vi "mqtt client server.vi"(6 "keep connected":refnum<vi>, 8 "connect success reference":refnum<vi>, 9 "mqtt prefix":string, 10 "client or server":enum16{"client", "server"}(ring), 11 "subsystem":string) -> (0 "error out":errorcluster)   [LabVIEW 2017]
uses:
  mqtt-LabVIEW/src/class/mqtt/mqttTypedef/mqttBroker.ctl
  mqtt-LabVIEW/src/class/mqtt/mqttTypedef/mqttConnectionFlags.ctl
  mqtt-LabVIEW/src/class/mqtt/mqttTypedef/mqttUserInformation.ctl
  mqtt-LabVIEW/src/class/mqtt/mqttTypedef/mqttWillInformation.ctl
  mqtt-LabVIEW/src/class/mqtt/mqttConfigFunction.ctl
  mqtt-LabVIEW/src/class/mqtt/mqttTXqueue/mqttTXdataQueueFunction.ctl
  mqtt-LabVIEW/src/class/mqtt/mqtt.lvclass
panel:
  out "connect success":bool
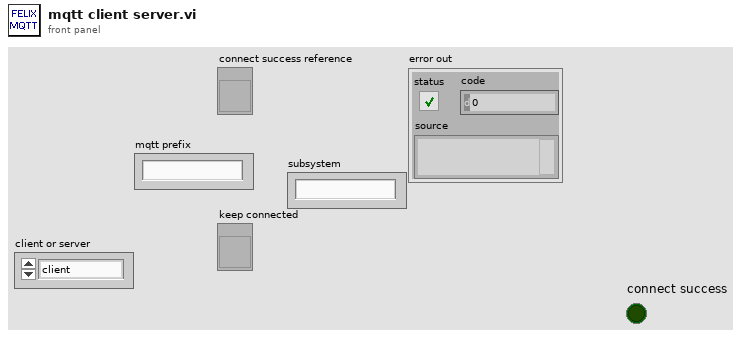
[diagram p1: front panel]
types:
  T1 = typedef "mqttWillInformation.ctl" = cluster{"User Name":string, "Password":string}
  T2 = typedef "mqttUserInformation.ctl" = cluster{"Will message":string, "Will Topic":string}
  T3 = typedef "mqttConnectionFlags.ctl" = cluster{"reserved":bool, "clean session":bool, "will flag":bool, "willQOS":enum8{"At most once", "At least once", "Exactly once", "Reserved"}, "will retain":bool, "password":bool, "user name":bool}
  T4 = typedef "mqttBroker.ctl" = cluster{"address":string, "port":u16, "connTimeout":i32, "writeTimeout":i32, "readTimeout":i32, "subTimeout":i32}
  T5 = typedef "mqttTXdataQueueFunction.ctl" = enum16{"init", "deinit", "getQueue", "enqueue"}
  T6 = typedef "mqtt.lvclass/mqttConfigFunction.ctl" = enum16{"init", "deinit", "set", "get"}
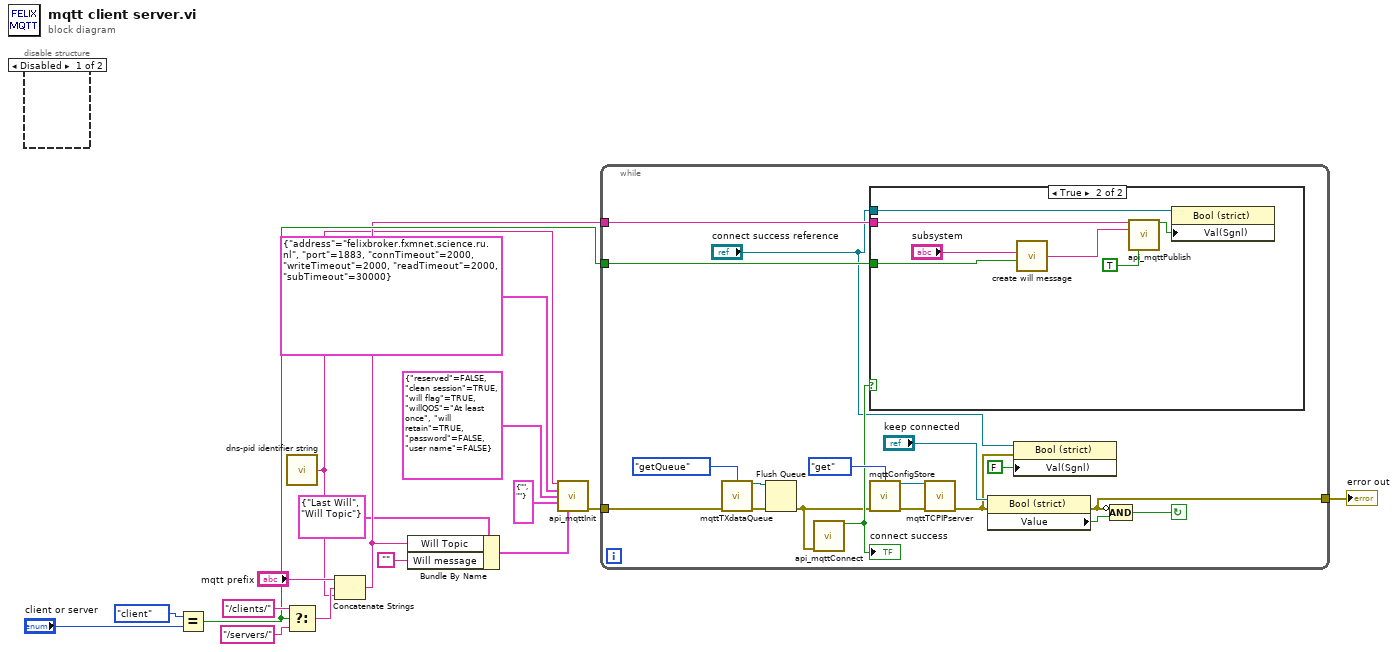
[diagram p0: block diagram]
diagram:
  n1 = disable-structure shown="Disabled" {
    frame Disabled {
    }
    frame Enabled {
    }
  }
  n2 = Equal?(x=enum16{"client", "server"}."client", y="client or server") -> (x = y?=w11:bool)
  n3 = call "dns-pid identifier string.vi"() -> ("DNS_PID Identifier string"=w1:string)  [unwired: 1 in]
  n4 = Select(t="/clients/" ("string"), s=w11, f="/servers/" ("string")) -> (s? t:f=w17:string)
  n5 = Concatenate Strings("mqtt prefix", w17, w1) -> (w10:string)
  n6 = Bundle By Name(cluster=T2 {"Will message"="Last Will", "Will Topic"="Will Topic"} ("Will Info"), "Will Topic"=w10, "Will message"="") -> (w3:T2)
  n7 = call "api_mqttInit.vi"("client"=w1, "broker"=T4 {"address"="felixbroker.fxmnet.science.ru.nl", "port"=1883, "connTimeout"=2000, "writeTimeout"=2000, "readTimeout"=2000, "subTimeout"=30000}, "connFlags"=T3 {"reserved"=FALSE, "clean session"=TRUE, "will flag"=TRUE, "willQOS"=enum."At least once", "will retain"=TRUE, "password"=FALSE, "user name"=FALSE}, "User Info"=T1 {"User Name"="", "Password"=""}, "Will Info"=w3) -> ("error out"=w2:errorcluster)  [unwired: 10 in]
  n8 = while {
    tunnel: w11 -> [w31]
    tunnel: w10 -> [w30]
    tunnel: [w29] -> w9
    tunnel: w2 -> [w19]
    stop <- w23 continue-if-true
    n9 = call "mqttTXdataQueue.vi"("function"=mqttTXdataQueueFunction."getQueue", "error in (no error)"=w19) -> ("Queue out"=w22:refnum<queue>, "error out"=w20:errorcluster)  [unwired: 12 in]
    n10 = Flush Queue(queue=w22, error in (no error)=w20) -> (error out=w18:errorcluster)  [unwired: 2 out]
    n11 = call "api_mqttConnect.vi"("error in (no error)"=w18) -> ("success"=w32:bool)  [unwired: 11 in, 3 out]
    "connect success" <- w32
    n12 = case shown="True" w32 {
      tunnel: w31 -> [_ w40]
      tunnel: w30 -> [_ w39]
      tunnel: "connect success reference" -> [_ w36]
      frame False {
      }
      frame True {
        n13 = call "create will message.vi"("client?"=w40, "subsystem"="subsystem") -> ("JSON string"=w42:string)  [unwired: 2 in]
        n14 = call "api_mqttPublish.vi"("topic"=w39, "value"=w42, "retain(F)"=TRUE) -> ("success"=w38:bool)  [unwired: 11 in, 1 out]
        n15 = property class="Bool (strict)"(reference=w36, "Val(Sgnl)"=w38) -> ()  [unwired: 1 in, 2 out]
      }
    }
    n16 = call "mqttConfigStore.vi"("function"=mqttConfigFunction."get", "error in (no error)"=w18) -> ("mqtt.lvclass out"=w35:refnum<class "mqtt.lvclass">, "error out"=w33:errorcluster)  [unwired: 12 in]
    n17 = call "mqttTCPIPserver.vi"("mqtt.lvclass"=w35, "error in (no error)"=w33) -> ("error out"=w25:errorcluster)  [unwired: 12 in, 1 out]
    n18 = property class="Bool (strict)"(reference="keep connected", error in=w25) -> (error out=w29:errorcluster, "Value"=w26:bool)  [unwired: 1 out]
    n19 = property class="Bool (strict)"(reference="connect success reference", error in=w25, "Val(Sgnl)"=FALSE ("Value (Signaling)")) -> ()  [unwired: 2 out]
    n20 = Compound Arithmetic op=AND(invert w29, w26) -> (w23:bool)
  }
  "error out" <- w9
